vi "Fixed Time Table Read.vi"(8 "error in":errorcluster, 9 "Data to read in":T2, 10 "Channel_Timing in":T1, 11 "Report Viewer in":refnum<class "Report Viewer.lvclass">) -> (0 "error out":errorcluster, 1 "Data to read out":T2, 2 "Channel_Timing out":T1, 3 "Report Viewer out":refnum<class "Report Viewer.lvclass">, 4 "Table Data":string[](array[string]), 6 "Table_Header":string[](array[string]))   [LabVIEW 2023, in "Report Viewer.lvlib" / "Report Viewer.lvclass"]
uses:
  Library/Report Viewer.lvclass
  Custom Controls/Data to Read.ctl
  Custom Controls/Channel_Timing.ctl
  Library/Report Viewer.lvclass/Report Viewer.ctl
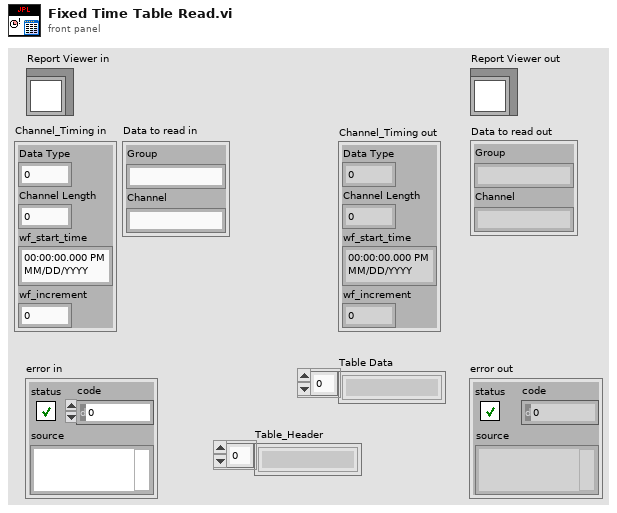
[diagram p1: front panel]
types:
  T1 = typedef "Report Viewer.lvlib/Report Viewer.lvclass/Channel_Timing.ctl" = cluster{"Data Type":u16, "Channel Length":u64, "wf_start_time":timestamp, "wf_increment":dbl}
  T2 = typedef "Report Viewer.lvlib/Report Viewer.lvclass/Data to Read.ctl" = cluster{"Group":string, "Channel":string}
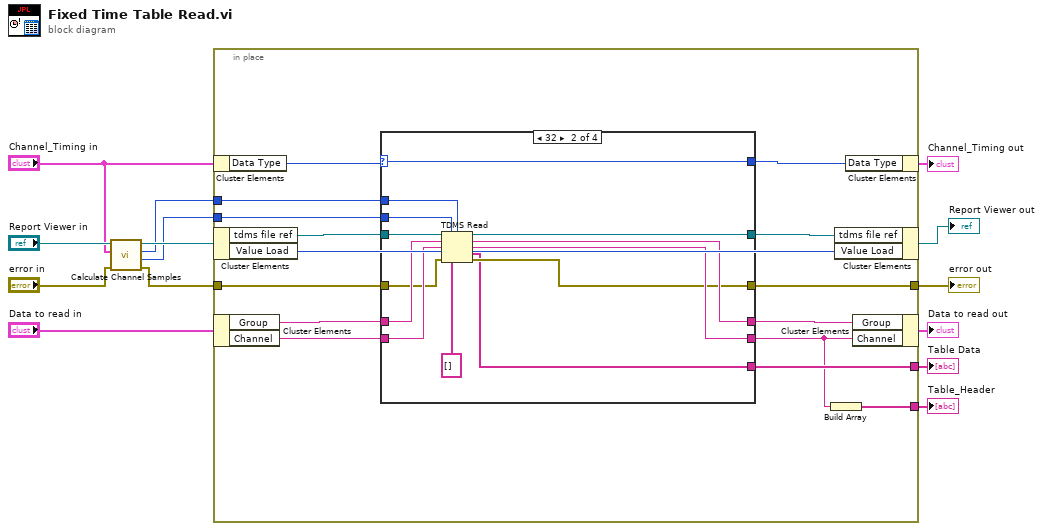
[diagram p0: block diagram]
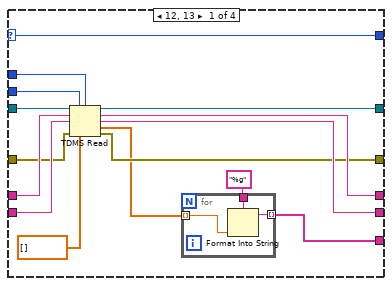
[diagram p2: hidden frame]
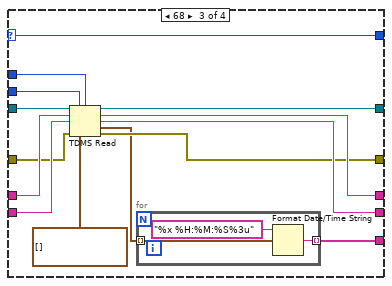
[diagram p3: hidden frame]
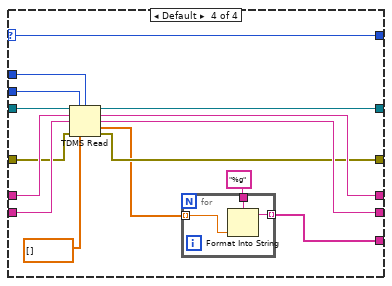
[diagram p4: hidden frame]
diagram:
  n1 = call "Calculate Channel Samples.vi"("error in"="error in", "Channel Timing"="Channel_Timing in", "Report Viewer in"="Report Viewer in") -> ("error out"=w5:errorcluster, "Sample Offset"=w1:u32, "Num_Samples"=w2:u32, "Report Viewer out"=w4:refnum<class "Report Viewer.lvclass">)  [unwired: 5 in]
  n2 = in-place {
    in-place-border: w5 -> [w22]
    in-place-border: [w20] -> w12
    in-place-border: [w19] -> w11
    in-place-border: [w17] -> w8
    in-place-border: w2 -> [w16]
    in-place-border: w1 -> [w15]
    n3 = in-place-cluster #1("Channel_Timing in") -> ("Data Type"=w28:u16)
    n4 = in-place-cluster #2(w4) -> ("tdms file ref"=w29:refnum<k34>, "Value Load"=w26:enum32{"Load All", "Load Selected"})
    n5 = in-place-cluster #3("Data to read in") -> ("Group"=w25:string, "Channel"=w24:string)
    n6 = case shown="32" w28 {
      selector: w28 -> [w43 w59 w73 w91]
      tunnel: w29 -> [w44 w60 w74 w92]
      tunnel: [w43 w59 w73 w91] -> w27
      tunnel: [w42 w58 w72 w90] -> w21
      tunnel: w25 -> [w41 w57 w71 w89]
      tunnel: w24 -> [w40 w56 w70 w88]
      tunnel: [w39 w55 w69 w87] -> w23
      tunnel: [w38 w54 w68 w86] -> w18
      tunnel: w22 -> [w37 w53 w67 w85]
      tunnel: [w36 w52 w66 w84] -> w20
      tunnel: [w33 w50 w63 w80] -> w19
      tunnel: w15 -> [w30 w48 w61 w78]
      tunnel: w16 -> [w31 w49 w62 w79]
      frame 12, 13 {
        n7 = TDMS Read(0:w44, 1:w30, 2:w31, 5:w41, 7:w40, 11:w37, 12:cdb[] []) -> (4:w42:refnum<k34>, 6:w39:string, 8:w38:string, 10:w34:cdb[], 15:w36:errorcluster)  [unwired: 1 in, 1 out]
        n8 = for {
          tunnel: "%g" ("format string") -> [w47]
          tunnel: w34 -> [w46] mode=indexing
          tunnel: [w45] -> w33 mode=indexing
          n9 = Format Into String(format string=w47, w46) -> (resulting string=w45:string)  [unwired: 2 in, 1 out]
        }
      }
      frame 32 {
        n10 = TDMS Read(0:w60, 1:w48, 2:w49, 5:w57, 7:w56, 11:w53, 12:string[] []) -> (4:w58:refnum<k34>, 6:w55:string, 8:w54:string, 10:w50:string[], 15:w52:errorcluster)  [unwired: 1 in, 1 out]
      }
      frame 68 {
        n11 = TDMS Read(0:w74, 1:w61, 2:w62, 5:w71, 7:w70, 11:w67, 12:timestamp[] []) -> (4:w72:refnum<k34>, 6:w69:string, 8:w68:string, 10:w64:timestamp[], 15:w66:errorcluster)  [unwired: 1 in, 1 out]
        n12 = for {
          tunnel: [w77] -> w63 mode=indexing
          tunnel: w64 -> [w76] mode=indexing
          n13 = Format Date/Time String(time format string (%c)="%x %H:%M:%S%3u", seconds (now)=w76) -> (date/time string=w77:string)  [unwired: 1 in]
        }
      }
      frame Default {
        n14 = TDMS Read(0:w92, 1:w78, 2:w79, 5:w89, 7:w88, 11:w85, 12:dbl[] []) -> (4:w90:refnum<k34>, 6:w87:string, 8:w86:string, 10:w81:dbl[], 15:w84:errorcluster)  [unwired: 1 in, 1 out]
        n15 = for {
          tunnel: "%g" ("format string") -> [w95]
          tunnel: w81 -> [w94] mode=indexing
          tunnel: [w93] -> w80 mode=indexing
          n16 = Format Into String(format string=w95, w94) -> (resulting string=w93:string)  [unwired: 2 in, 1 out]
        }
      }
    }
    n17 = Build Array(w18) -> (w17:string[])
    n18 = in-place-cluster #2("tdms file ref"=w21, "Value Load"=w26) -> (→"Report Viewer out":refnum<class "Report Viewer.lvclass">)
    n19 = in-place-cluster #1("Data Type"=w27) -> (→"Channel_Timing out":T1)
    n20 = in-place-cluster #3("Group"=w23, "Channel"=w18) -> (→"Data to read out":T2)
  }
  "error out" <- w12
  "Table Data" <- w11
  "Table_Header" <- w8
